vi "Start_Simulation_Engine.vi"(11 "error in":errorcluster) -> (15 "error out":errorcluster)   [LabVIEW 2017]
doc: "Sets a reference into a registry, gets a reference from a registry, or deletes a reference from a registry. The reference is accessed by name, and can be given any unique name.\n\nThis software is licensed. Open the labview\\readme\\WPI Robotics Library Open Source License.txt file for more information."
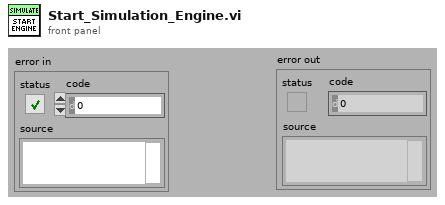
[diagram p1: front panel]
types:
  T1 = enum32{"Bad", "Idle", "Run top level", "Running"}
  T2 = typedef "LVRectTypeDef.ctl" = cluster{"Left":i16, "Top":i16, "Right":i16, "Bottom":i16}
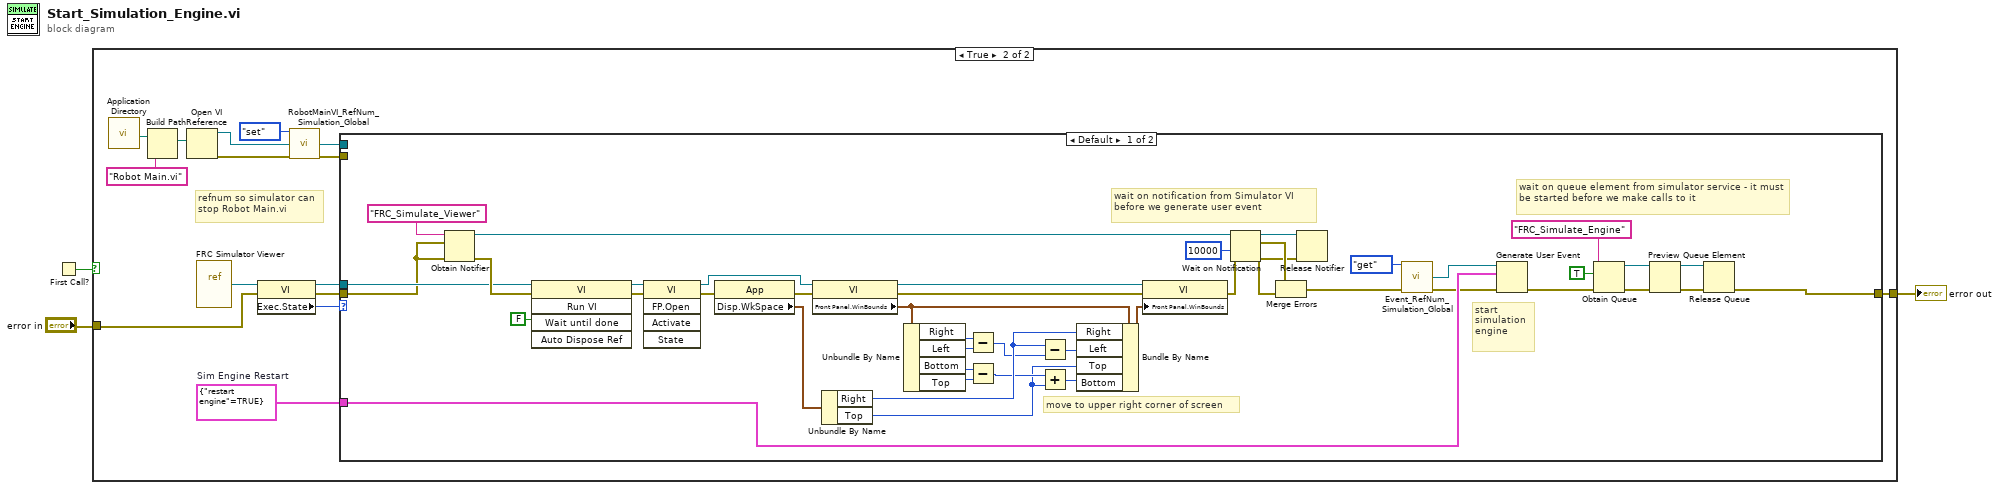
[diagram p0: block diagram]
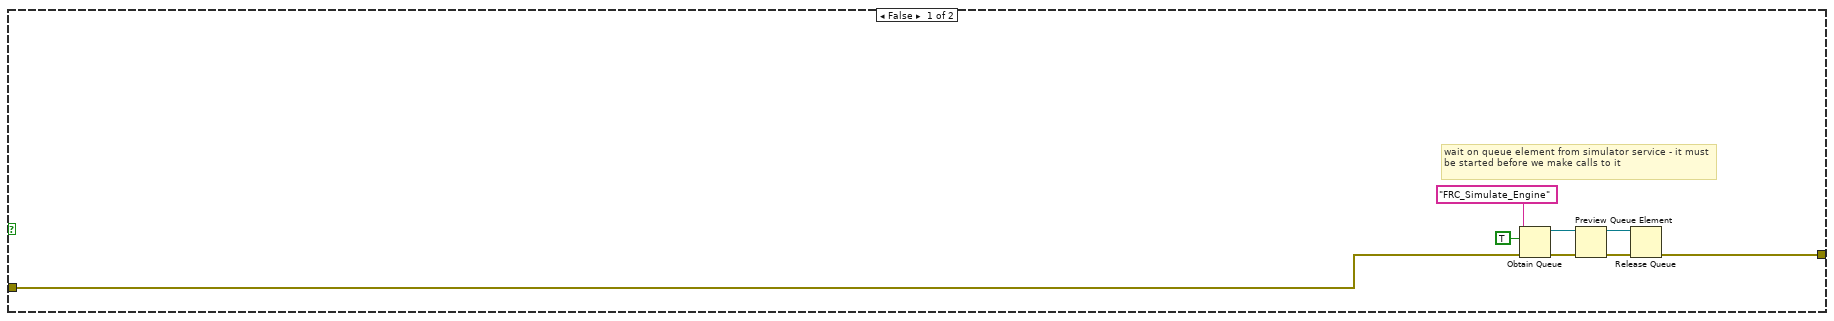
[diagram p2: hidden frame]
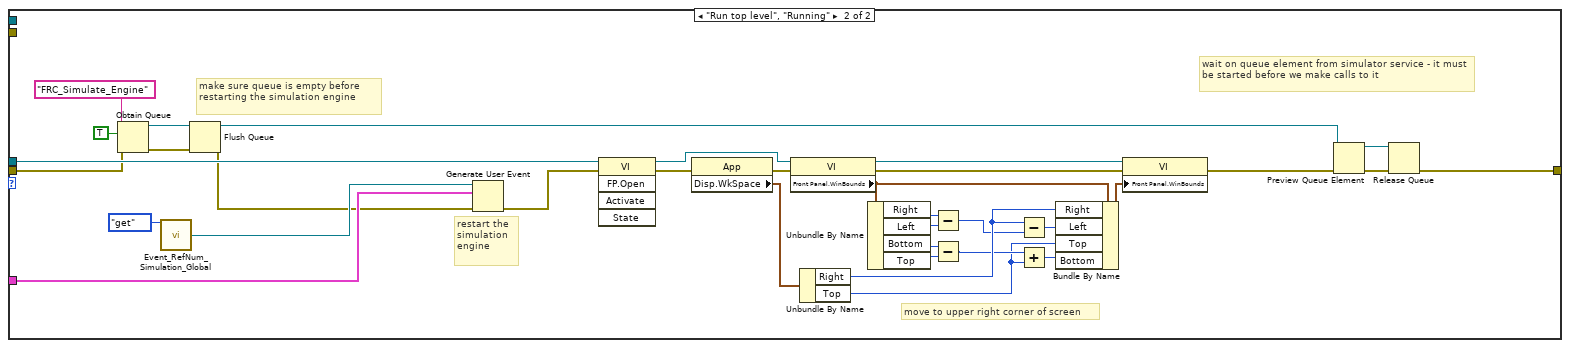
[diagram p3: hidden frame]
diagram:
  n1 = First Call?() -> (First Call?: T/F=w2:bool)
  n2 = case shown="True" w2 {
    tunnel: [w4 w23] -> w3
    tunnel: "error in" -> [w5 w21]
    frame False {
      # "wait on queue element from simulator service - it must be started before we make calls to it"
      n3 = Obtain Queue(name (unnamed)="FRC_Simulate_Engine", element data type=TRUE ("loop on"), error in (no error)=w5) -> (queue out=w11:refnum<queue>, error out=w10:errorcluster)  [unwired: 2 in, 1 out]
      n4 = Preview Queue Element(queue=w11, error in (no error)=w10) -> (queue out=w6:refnum<queue>, error out=w7:errorcluster)  [unwired: 1 in, 2 out]
      n5 = Release Queue(queue=w6, error in (no error)=w7) -> (error out=w4:errorcluster)  [unwired: 1 in, 2 out]
    }
    frame True {
      w20 = cluster{"restart engine":bool} {"restart engine"=TRUE}  # Sim Engine Restart
      # "refnum so simulator can stop Robot Main.vi"
      n6 = call <vilib>:"Application Directory.vi"() -> ("Application Directory"=w15:path)
      n7 = Build Path(base path=w15, name or relative path="Robot Main.vi") -> (appended path=w16:path)
      n8 = Open VI Reference(vi path=w16) -> (vi reference=w17:refnum<vi>, error out=w13:errorcluster)  [unwired: 5 in]
      n9 = vi-ref <vilib>:"FRC Simulator Viewer.vi"() -> (w22:refnum<vi>)
      n10 = property class="VI"(reference=w22, error in=w21) -> (reference out=w24:refnum<vi>, error out=w25:errorcluster, "Exec.State"=w26:T1)
      n11 = call <vilib>:"RobotMainVI_RefNum_Simulation_Global.vi"("menu"=enum16{"set", "get", "delete"}."set", "VI Refnum in"=w17, "error in (no error)"=w13) -> ("VI Refnum out"=w12:refnum<vi>, "error out"=w18:errorcluster)  [unwired: 11 in]
      n12 = case shown="Default" w26 {
        tunnel: w25 -> [w38 w76]
        tunnel: w24 -> [w39 w84]
        tunnel: [w28 w77] -> w23
        tunnel: w20 -> [w42 w86]
        tunnel: w18 -> [_ _]
        tunnel: w12 -> [_ _]
        frame Default {
          # "wait on notification from Simulator VI before we generate user event"
          # "start simulation engine"
          # "wait on queue element from simulator service - it must be started before we make calls to it"
          # "move to upper right corner of screen"
          n13 = Obtain Notifier(name (unnamed)="FRC_Simulate_Viewer", notification data type=w38, error in (no error)=w38) -> (notifier out=w48:refnum<notifier>, error out=w40:errorcluster)  [unwired: 1 in, 1 out]
          n14 = invoke class="VI" method="Run VI"(reference=w39, error in=w40, "Wait until done"=FALSE ("Wait Until Done")) -> (reference out=w69:refnum<vi>, error out=w68:errorcluster)  [unwired: 2 in, 3 out]
          n15 = invoke class="VI" method="FP.Open"(reference=w69, error in=w68) -> (reference out=w67:refnum<vi>, error out=w66:errorcluster)  [unwired: 3 in, 3 out]
          n16 = property class="App"(error in=w66) -> (error out=w64:errorcluster, "Disp.WkSpace"=w65:T2)  [unwired: 1 in, 1 out]
          n17 = property class="VI"(reference=w67, error in=w64) -> (reference out=w61:refnum<vi>, error out=w63:errorcluster, "Front Panel.WinBounds"=w60:T2)
          n18 = Unbundle By Name(w65) -> ("Right"=w56:i16, "Top"=w50:i16)
          n19 = Unbundle By Name(w60) -> ("Right"=w59:i16, "Left"=w58:i16, "Bottom"=w53:i16, "Top"=w54:i16)
          n20 = Subtract(x=w59, y=w58) -> (x-y=w55:i16)
          n21 = Subtract(x=w53, y=w54) -> (x-y=w51:i16)
          n22 = Subtract(x=w56, y=w55) -> (x-y=w57:i16)
          n23 = Add(x=w51, y=w50) -> (x+y=w52:i16)
          n24 = Bundle By Name(cluster=w60, "Right"=w56, "Left"=w57, "Top"=w50, "Bottom"=w52) -> (w62:T2)
          n25 = property class="VI"(reference=w61, error in=w63, "Front Panel.WinBounds"=w62) -> (error out=w46:errorcluster)  [unwired: 1 out]
          n26 = Wait on Notification(notifier=w48, timeout in ms (-1)=10000, error in (no error)=w46) -> (notifier out=w45:refnum<notifier>, notification=w47:errorcluster, error out=w44:errorcluster)  [unwired: 1 in, 1 out]
          n27 = Merge Errors(w47, w44) -> (w37:errorcluster)
          n28 = Release Notifier(notifier=w45, error in (no error)=w44) -> ()  [unwired: 1 in, 3 out]
          n29 = call <vilib>:"Event_RefNum_Simulation_Global.vi"("menu"=enum16{"set", "get", "delete"}."get", "error in (no error)"=w37) -> ("FRC_Sim_Events out"=w35:refnum<user-event>, "error out"=w36:errorcluster)  [unwired: 12 in]
          n30 = Generate User Event(user event=w35, event data cluster=w42, error in=w36) -> (error out=w31:errorcluster)  [unwired: 1 in, 1 out]
          n31 = Obtain Queue(name (unnamed)="FRC_Simulate_Engine", element data type=TRUE ("loop on"), error in (no error)=w31) -> (queue out=w34:refnum<queue>, error out=w33:errorcluster)  [unwired: 2 in, 1 out]
          n32 = Preview Queue Element(queue=w34, error in (no error)=w33) -> (queue out=w27:refnum<queue>, error out=w29:errorcluster)  [unwired: 1 in, 2 out]
          n33 = Release Queue(queue=w27, error in (no error)=w29) -> (error out=w28:errorcluster)  [unwired: 1 in, 2 out]
        }
        frame "Run top level", "Running" {
          # "make sure queue is empty before restarting the simulation engine"
          # "wait on queue element from simulator service - it must be started before we make calls to it"
          # "restart the simulation engine"
          # "move to upper right corner of screen"
          n34 = Obtain Queue(name (unnamed)="FRC_Simulate_Engine", element data type=TRUE ("loop on"), error in (no error)=w76) -> (queue out=w73:refnum<queue>, error out=w75:errorcluster)  [unwired: 2 in, 1 out]
          n35 = call <vilib>:"Event_RefNum_Simulation_Global.vi"("menu"=enum16{"set", "get", "delete"}."get") -> ("FRC_Sim_Events out"=w82:refnum<user-event>)  [unwired: 13 in, 1 out]
          n36 = Flush Queue(queue=w73, error in (no error)=w75) -> (queue out=w71:refnum<queue>, error out=w74:errorcluster)  [unwired: 1 out]
          n37 = Generate User Event(user event=w82, event data cluster=w86, error in=w74) -> (error out=w85:errorcluster)  [unwired: 1 in, 1 out]
          n38 = invoke class="VI" method="FP.Open"(reference=w84, error in=w85) -> (reference out=w104:refnum<vi>, error out=w103:errorcluster)  [unwired: 3 in, 3 out]
          n39 = property class="App"(error in=w103) -> (error out=w101:errorcluster, "Disp.WkSpace"=w102:T2)  [unwired: 1 in, 1 out]
          n40 = property class="VI"(reference=w104, error in=w101) -> (reference out=w98:refnum<vi>, error out=w100:errorcluster, "Front Panel.WinBounds"=w97:T2)
          n41 = Unbundle By Name(w102) -> ("Right"=w93:i16, "Top"=w87:i16)
          n42 = Unbundle By Name(w97) -> ("Right"=w96:i16, "Left"=w95:i16, "Bottom"=w90:i16, "Top"=w91:i16)
          n43 = Subtract(x=w96, y=w95) -> (x-y=w92:i16)
          n44 = Subtract(x=w90, y=w91) -> (x-y=w88:i16)
          n45 = Subtract(x=w93, y=w92) -> (x-y=w94:i16)
          n46 = Add(x=w88, y=w87) -> (x+y=w89:i16)
          n47 = Bundle By Name(cluster=w97, "Right"=w93, "Left"=w94, "Top"=w87, "Bottom"=w89) -> (w99:T2)
          n48 = property class="VI"(reference=w98, error in=w100, "Front Panel.WinBounds"=w99) -> (error out=w72:errorcluster)  [unwired: 1 out]
          n49 = Preview Queue Element(queue=w71, error in (no error)=w72) -> (queue out=w78:refnum<queue>, error out=w79:errorcluster)  [unwired: 1 in, 2 out]
          n50 = Release Queue(queue=w78, error in (no error)=w79) -> (error out=w77:errorcluster)  [unwired: 1 in, 2 out]
        }
      }
    }
  }
  "error out" <- w3
